vi "Sync Project Load Config.vi"(8 "Error In":errorcluster, 11 "Sync Source Config":T1) -> (0 "Error Out":errorcluster, 1 "Backup Path":path, 2 "Project Source Root Dir":path, 3 "Sync Source Config":T1)   [LabVIEW 2011, in "LVH-Build-Tools.lvlib"]
doc: "Load Sync Project configuration data from .ini"
uses:
  <vilib>/LabVIEW Hacker/Build Tools/LVH-Build-Tools.lvlib
  Type Defs/Sync Source Configuration.ctl
  Type Defs/Installed Project.ctl
  Local Toolbox/_Installed LabVIEW Version.ctl
  <vilib>/Utility/config.llb/Read Key (String).vi
  <vilib>/Utility/config.llb/NI_LVConfig.lvlib
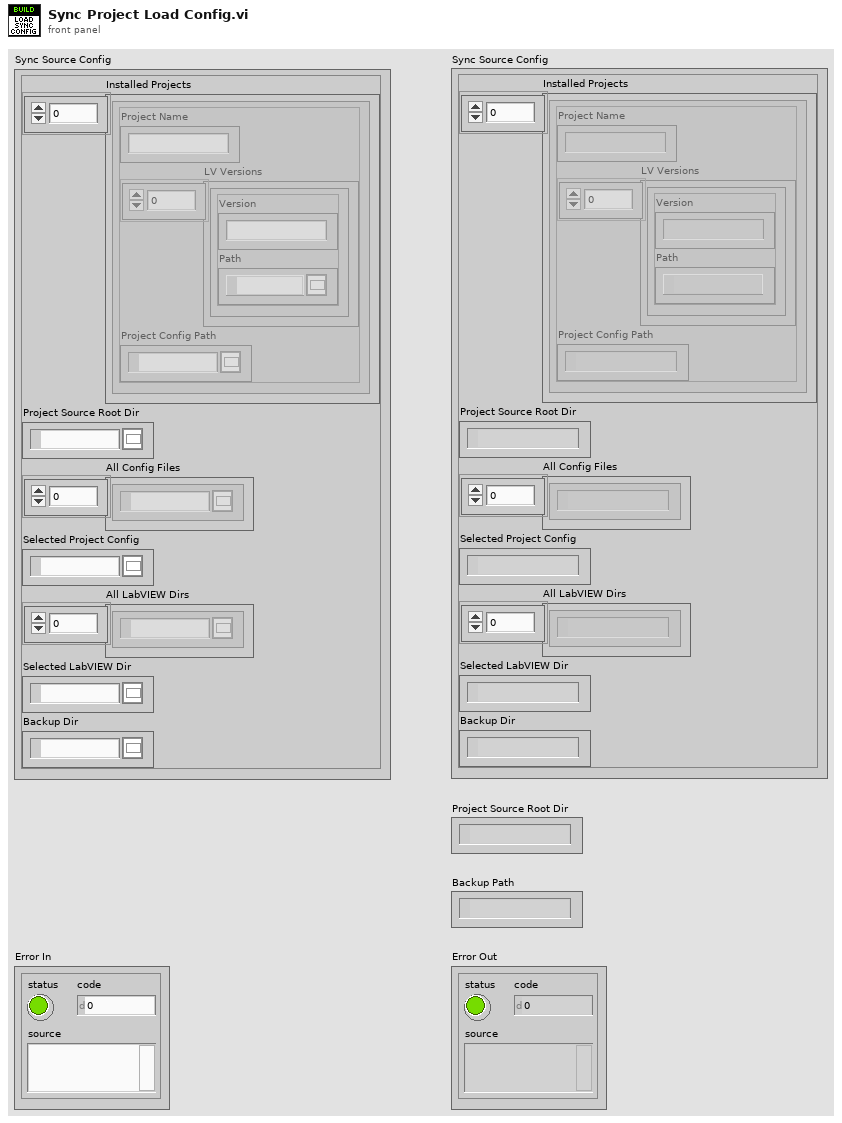
[diagram p1: front panel]
types:
  T1 = typedef "LVH-Build-Tools.lvlib/Sync Source Configuration.ctl" = cluster{"Installed Projects":T2[], "Project Source Root Dir":path, "All Config Files":path[], "Selected Project Config":path, "All LabVIEW Dirs":path[], "Selected LabVIEW Dir":path, "Backup Dir":path}
  T2 = typedef "LVH-Build-Tools.lvlib/Installed Project.ctl" = cluster{"Project Name":string, "LV Versions":T3[], "Project Config Path":path}
  T3 = typedef "LVH-Build-Tools.lvlib/_Installed LabVIEW Version.ctl" = cluster{"Version":string, "Path":path}
  T4 = typedef "NI_LVConfig.lvlib/Config Data RefNum.ctl" = refnum<k1>
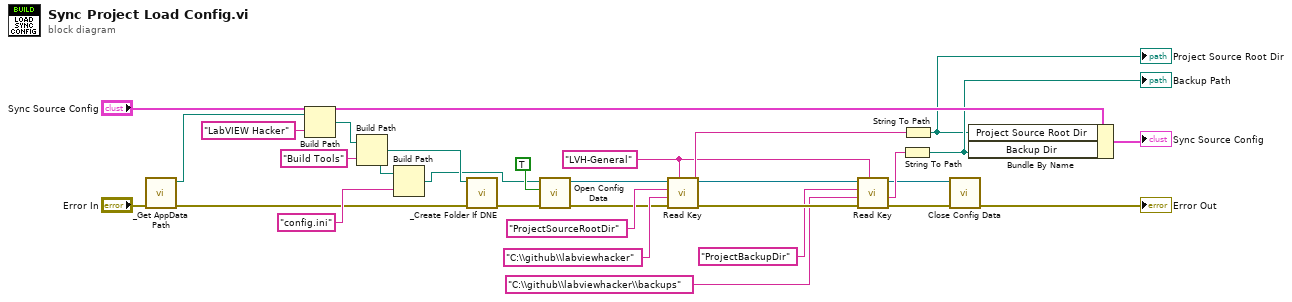
[diagram p0: block diagram]
diagram:
  w15 = "LVH-General" ("section")
  n1 = call "_Get AppData Path.vi"("Error In"="Error In") -> ("Error Out"=w4:errorcluster, "LabVIEW Data Path"=w6:path)  [unwired: 9 in]
  n2 = Build Path(base path=w6, name or relative path="LabVIEW Hacker") -> (appended path=w7:path)
  n3 = Build Path(base path=w7, name or relative path="Build Tools") -> (appended path=w2:path)
  n4 = Build Path(base path=w2, name or relative path="config.ini" ("string")) -> (appended path=w1:path)
  n5 = call "_Create Folder If DNE.vi"("Error In"=w4, "Folder Path"=w2) -> ("Error Out"=w3:errorcluster)  [unwired: 8 in, 1 out]
  n6 = call <vilib>:"Open Config Data.vi"("error in (no error)"=w3, "create file if necessary (T)"=TRUE, "configuration file path"=w1) -> ("error out"=w19:errorcluster, "refnum"=w20:T4)  [unwired: 6 in, 1 out]
  n7 = call-poly <vilib>:"Read Key.vi"("section"=w15, "error in (no error)"=w19, "default value"="C:\\github\\labviewhacker", "key"="ProjectSourceRootDir", "refnum"=w20) -> ("error out"=w27:errorcluster, "value"=w28:string, "refnum out"=w26:T4)  [unwired: 3 in, 1 out]
  n8 = call-poly <vilib>:"Read Key.vi"("section"=w15, "error in (no error)"=w27, "default value"="C:\\github\\labviewhacker\\backups", "key"="ProjectBackupDir", "refnum"=w26) -> ("error out"=w18:errorcluster, "value"=w23:string, "refnum out"=w17:T4)  [unwired: 3 in, 1 out]
  n9 = String To Path(string=w23) -> (path=w14:path)
  "Backup Path" <- w14
  n10 = String To Path(string=w28) -> (path=w13:path)
  "Project Source Root Dir" <- w13
  n11 = call <vilib>:"Close Config Data.vi"("error in (no error)"=w18, "refnum"=w17) -> ("error out"=→"Error Out":errorcluster)  [unwired: 8 in, 1 out]
  n12 = Bundle By Name(cluster="Sync Source Config", "Project Source Root Dir"=w13, "Backup Dir"=w14) -> (→"Sync Source Config":T1)
